vi "Parse All Notes.vi"(8 "error in (no error)":errorcluster, 10 "SR Cluster in":T1 {"Creation Date" format="%<%x>T"; "Last Updated" format="%<%x>T"}, 11 "result string":string) -> (0 "error out":errorcluster, 2 "SR Cluster out":T1 {"Creation Date" format="%<%x>T"; "Last Updated" format="%<%x>T"}, 3 "Array":T3[](array[typedef]) {"Note Date" format="%<%x >T"})   [LabVIEW 2018]
uses:
  Type Defs/SR Note Cluster.ctl
  Type Defs/SR Cluster.ctl
  Type Defs/SR Status.ctl
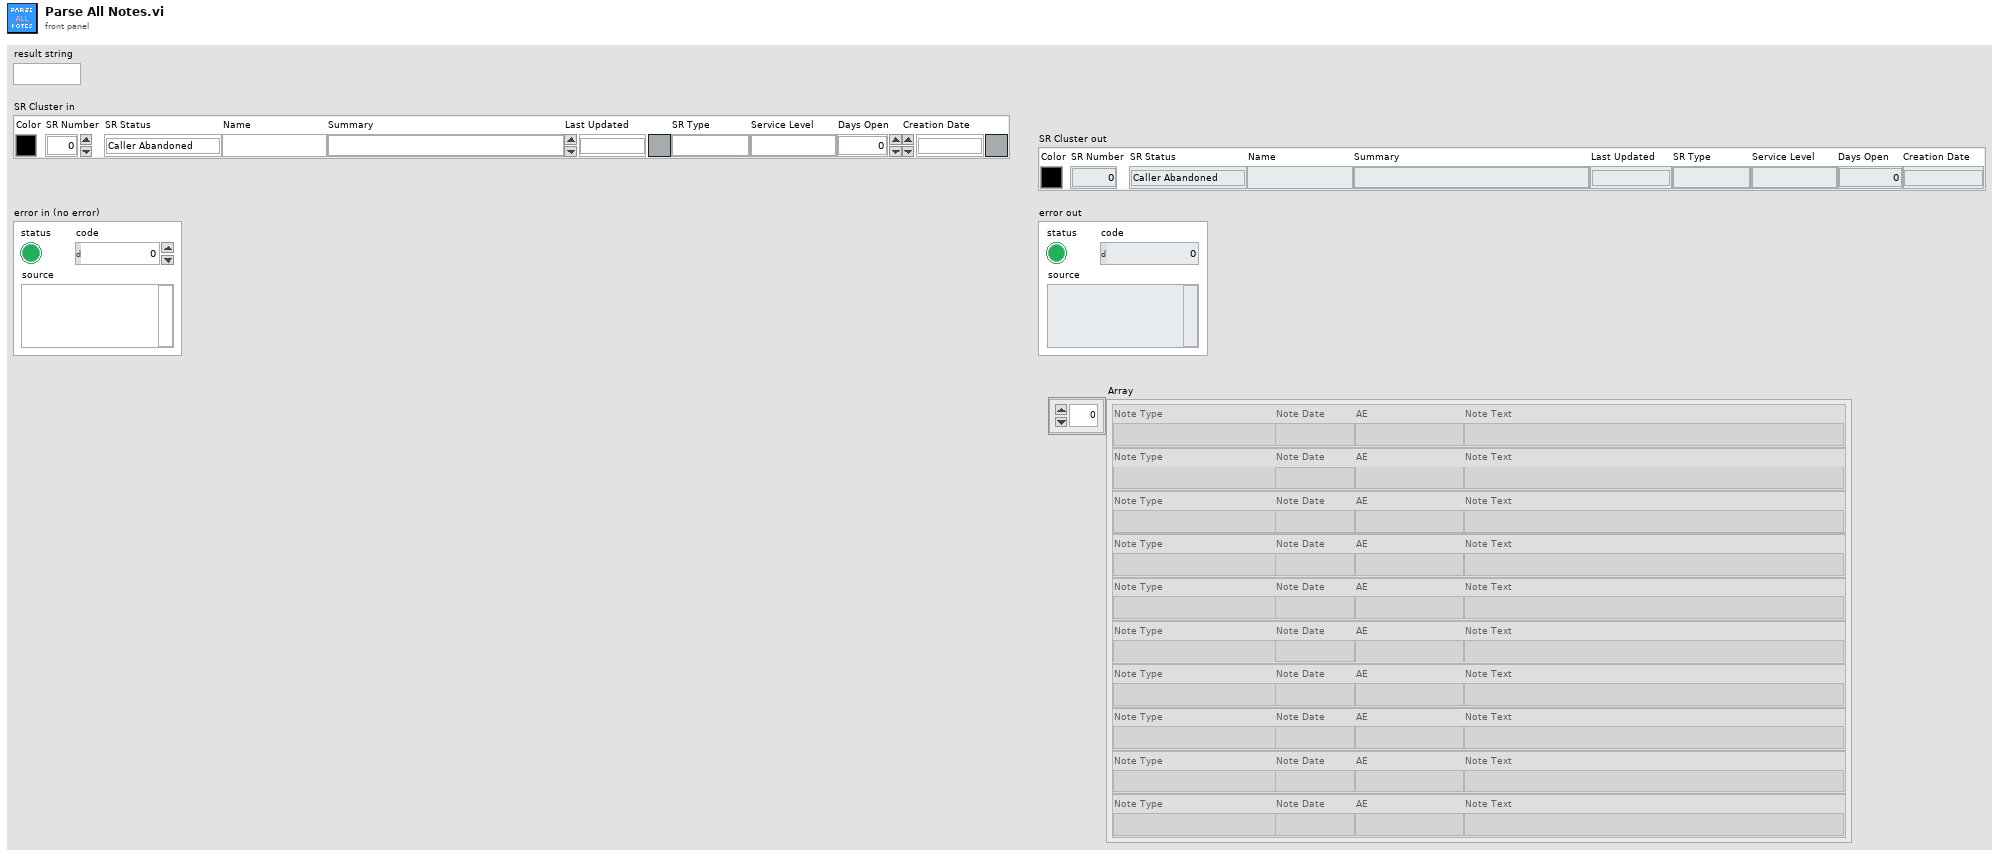
[diagram p1: front panel]
types:
  T1 = typedef "SR Cluster.ctl" = cluster{"Color":u32, "SR Number":i32, "SR Status":T2, "Name":string, "Summary":string, "Last Updated":timestamp, "SR Type":string, "Service Level":string, "Days Open":dbl, "Creation Date":timestamp}
  T2 = typedef "SR Status.ctl" = enum16{"Caller Abandoned", "Created in Error", "Expired", "Forum Resolved AE", "Forum Resolved Customer", "IN WORK", "IN WORK Collab with AES", "IN WORK Collab with PSE", "IN WORK Collab with SE", "IN WORK Customer Added Note", "IN WORK Escalation", "IN WORK Wait on Customer", "Open", "Potentially Resolved", "Presumed Resolved", "RMA Approved for Return", "Resolved", "Passed Off"}
  T3 = typedef "SR Note Cluster.ctl" = cluster{"Note Type":string, "Note Date":timestamp, "AE":string, "Note Text":string}
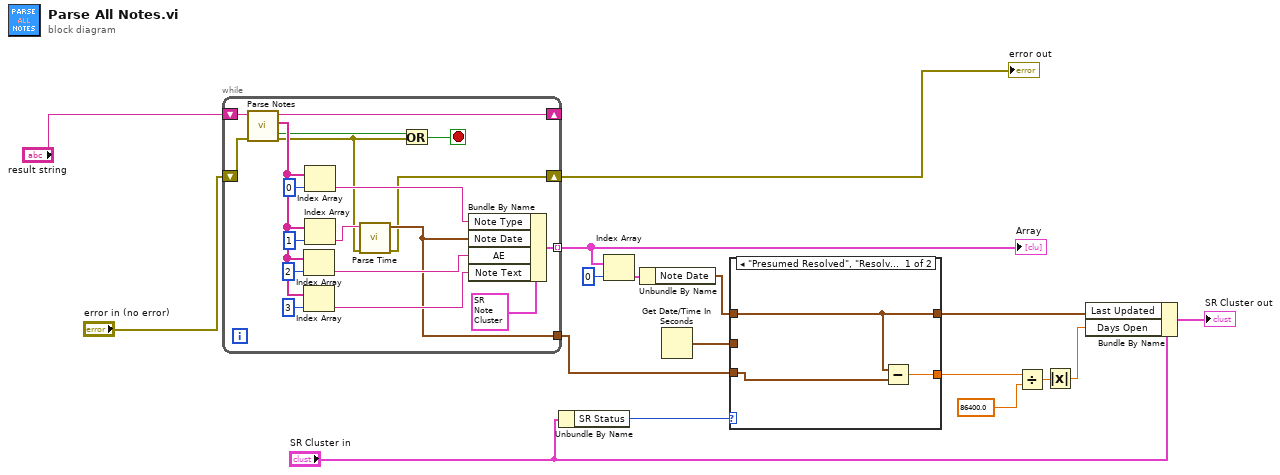
[diagram p0: block diagram]
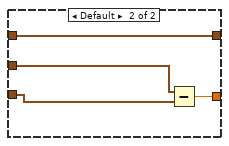
[diagram p2: hidden frame]
diagram:
  n1 = while {
    shift-right: [w35] -> _
    shift-left: "result string" -> [w36]
    tunnel: [w24] -> w11 mode=indexing
    tunnel: [w20] -> w9
    shift-right: [w19] -> w16
    shift-left: "error in (no error)" -> [w34]
    stop <- w23 stop-if-true
    n2 = call "Parse Notes.vi"("error in"=w34, "string in"=w36) -> ("error out"=w18:errorcluster, "Done Reading?"=w22:bool, "sr note out"=w33:string[], "result string out"=w35:string)  [unwired: 6 in]
    n3 = Index Array(array=w33, index=2) -> (element=w26:string)
    n4 = Index Array(array=w33, index=3) -> (element=w27:string)
    n5 = Index Array(array=w33, index=0) -> (element=w25:string)
    n6 = Index Array(array=w33, index=1) -> (element=w21:string)
    n7 = call "Parse Time.vi"("error in (no error)"=w18, "data"=w21) -> ("error out"=w19:errorcluster, "Time Stamp"=w20:timestamp)  [unwired: 8 in]
    n8 = Or(x=w22, y=w18) -> (x .or. y?=w23:bool)
    n9 = Bundle By Name(cluster=T3 {"Note Type"="", "Note Date"=timestamp(0 s since 1904-01-01), "AE"="", "Note Text"=""} ("SR Note Cluster"), "Note Type"=w25, "Note Date"=w20, "AE"=w26, "Note Text"=w27) -> (w24:T3)
  }
  "error out" <- w16
  "Array" <- w11
  n10 = Unbundle By Name("SR Cluster in") -> ("SR Status"=w10:T2)
  n11 = Index Array(array=w11, index=0) -> (element=w13:T3)
  n12 = Unbundle By Name(w13) -> ("Note Date"=w14:timestamp)
  n13 = Get Date/Time In Seconds() -> (seconds since 1Jan1904=w8:timestamp)
  n14 = case shown="\"Presumed Resolved\", \"Resolved\"" w10 {
    tunnel: w14 -> [w39 w40]
    tunnel: w9 -> [w37 w41]
    tunnel: w8 -> [_ w42]
    tunnel: [w38 w43] -> w2
    tunnel: [w39 w40] -> w1
    frame "Presumed Resolved", "Resolved" {
      n15 = Subtract(x=w39, y=w37) -> (x-y=w38:dbl)
    }
    frame Default {
      n16 = Subtract(x=w42, y=w41) -> (x-y=w43:dbl)
    }
  }
  n17 = Divide(x=w2, y=86400.0) -> (x/y=w5:dbl)
  n18 = Absolute Value(x=w5) -> (abs(x)=w3:dbl)
  n19 = Bundle By Name(cluster="SR Cluster in", "Last Updated"=w1, "Days Open"=w3) -> (→"SR Cluster out":T1)
